vi "ElevatorPIDFinalPlat.vi"(9 "Elevator Setpoint":dbl format="%.2f") -> (15 "At Setpoint":bool)   [LabVIEW 2014]
uses:
  Robot Global Data.vi
  <vilib>/addons/control/pid/pid.llb/PID (DBL).vi
  <vilib>/addons/control/pid/NI_PID_pid.lvlib
panel:
  out "Encoder Graph":dbl[](graph)
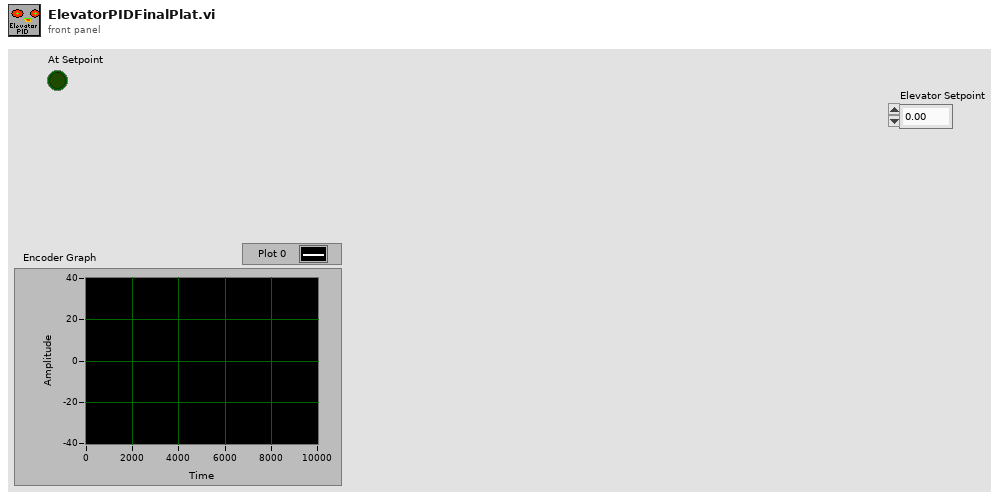
[diagram p1: front panel]
types:
  T1 = cluster{"proportional gain (Kc)":dbl, "integral time (Ti, min)":dbl, "derivative time (Td, min)":dbl}
  T2 = typedef "WPI_MotorControlDeviceRef.ctl" = cluster{"DeviceStatus":errorcluster, "Type":T3, "PWM":cluster{"Controller":T4, "PWM Channel":T5, "DeadBand":T6}, "CAN":cluster{"Device Number":u8, "Control Mode":T7, "Semaphore":T8, "Max Vout":dbl, "TalonSRX Control Mode":T9}, "Invert":bool, "TransformRef":T10, "InvTransformRef":T10}
  T3 = typedef "WPI_MotorControlType.ctl" = enum16{"PWM", "CAN", "CANTalonSRX"}
  T4 = typedef "FPGA_TypedefDigitalModule.ctl" = enum16{"Controller 1"}
  T5 = typedef "FPGA_DIOPWMChannel.ctl" = enum8{"PWM 0", "PWM 1", "PWM 2", "PWM 3", "PWM 4", "PWM 5", "PWM 6", "PWM 7", "PWM 8", "PWM 9", "PWM MXP 0", "PWM MXP 1", "PWM MXP 2", "PWM MXP 3", "PWM MXP 4", "PWM MXP 5", "PWM MXP 6", "PWM MXP 7", "PWM MXP 8", "PWM MXP 9", "Invalid"}
  T6 = typedef "WPI_PWMDeadband.ctl" = cluster{"Name":string, "maxPositivePwm":i32, "minPositivePwm":i32, "centerPwm":i32, "maxNegativePwm":i32, "minNegativePwm":i32, "angularRange":u16}
  T7 = typedef "WPI_CANJaguar_ControlMode.ctl" = enum8{"Percent VBus", "Current", "Speed", "Position", "Voltage"}
  T8 = typedef "Semaphore RefNum" = refnum<k1>
  T9 = typedef "WPI_CANTalonSRX_APIControlMode.ctl" = enum8{"Percent VBus", "Speed", "Position", "Slave", "Unchanged / Invalid"}
  T10 = typedef "WPI_PWMTransform_ConPane.ctl" = refnum<vi>
  T11 = typedef "WPI_CANTalonSRX_GlobalStatus.ctl" = cluster{"Applied Throttle":dbl, "Module Enabled":bool, "CAN Error":errorcluster, "Closed Loop Error":dbl, "Forward Limit Switch Closed":bool, "Reverse Limit Switch Closed":bool, "Sensor Position":dbl, "Sensor Velocity":dbl, "Current":dbl, "Sticky Fault - Over Temp":bool, "Sticky Fault - Under Voltage":bool, "Sticky Fault - Forward Limit":bool, "Sticky Fault - Reverse Limit":bool, "Sticky Fault - Forward Soft Limit":bool, "Sticky Fault - Reverse Soft Limit":bool, "Brake is Enabled":bool, "Encoder Position":dbl, "Encoder Velocity":dbl, "Encoder Index Count":dbl, "Encoder A Pin State":bool, "Encoder B Pin State":bool, "Encoder Index Pin State":bool, "Analog In":dbl, "Analog In Velocity":dbl, "Temperature (C)":dbl, "Battery Voltage":dbl}
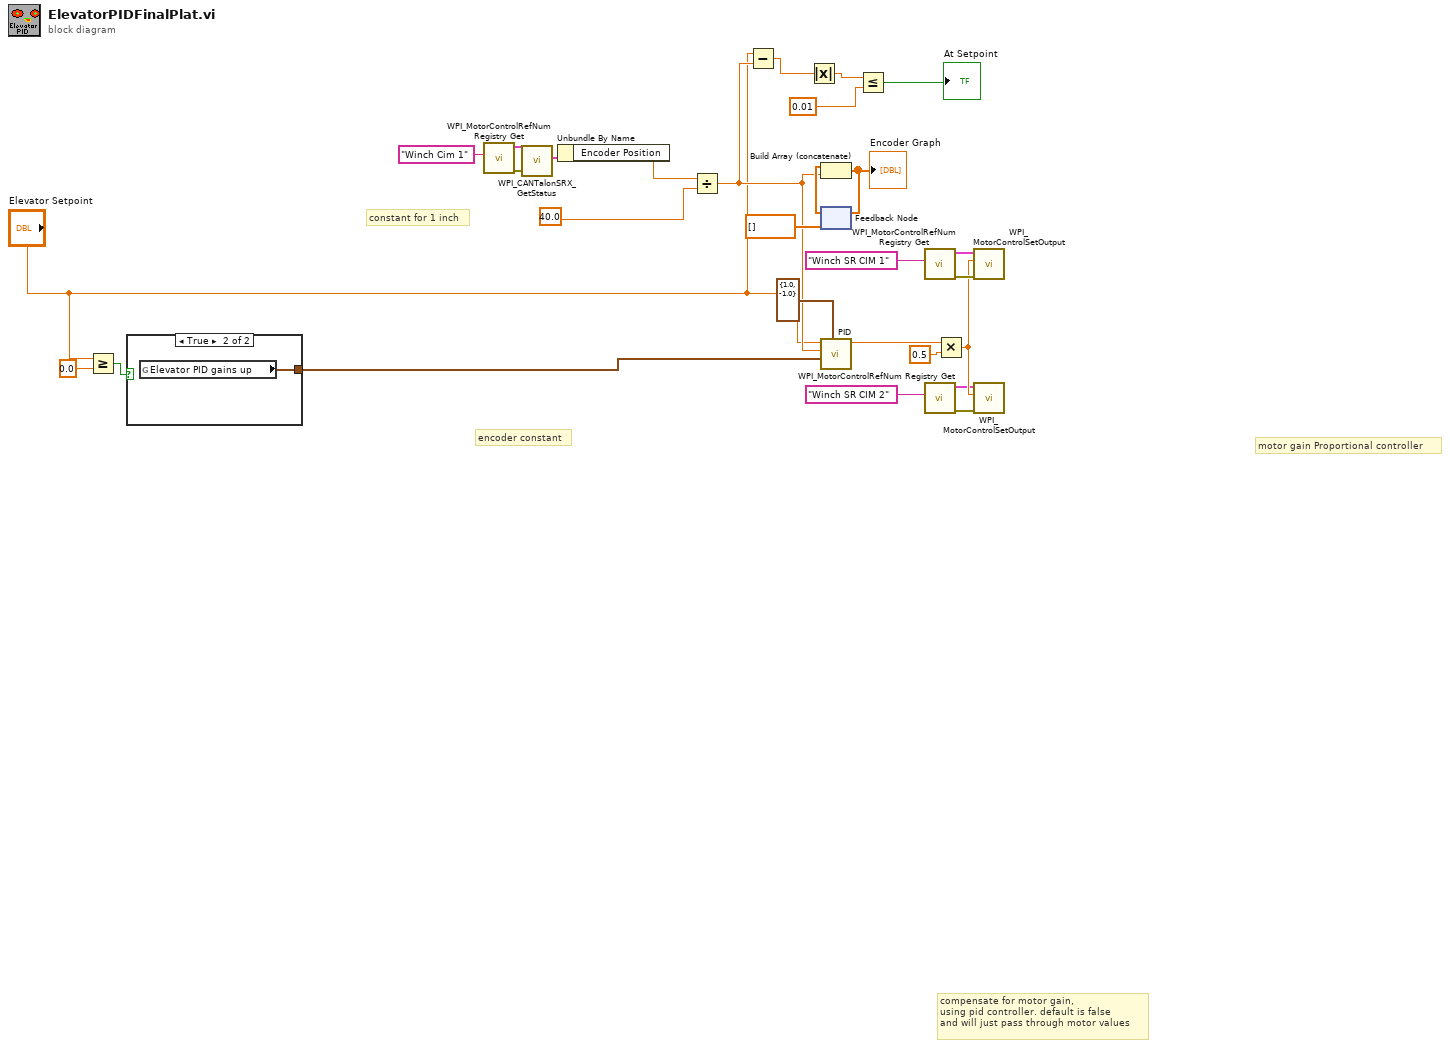
[diagram p0: block diagram]
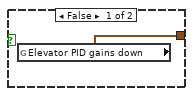
[diagram p2: hidden frame]
diagram:
  # "constant for 1 inch"
  # "encoder constant"
  # "motor gain Proportional controller"
  # "compensate for motor gain,\nusing pid controller. default is false\nand will just pass through motor values"
  n1 = Greater Or Equal?(x="Elevator Setpoint", y=0.0) -> (x >= y?=w16:bool)
  n2 = case shown="True" w16 {
    tunnel: [w29 w30] -> w27
    frame False {
      n3 = global read "Robot Global Data.vi" "Elevator PID gains down"() -> (w29:T1)
    }
    frame True {
      n4 = global read "Robot Global Data.vi" "Elevator PID gains up"() -> (w30:T1)
    }
  }
  n5 = call <vilib>:"WPI_MotorControlRefNum Registry Get.vi"("refnum name"="Winch Cim 1") -> ("error out"=w5:errorcluster, "MotorControlDevRef"=w4:T2)  [unwired: 9 in]
  n6 = call <vilib>:"WPI_CANTalonSRX_GetStatus.vi"("error in (no error)"=w5, "CAN Talon SRX Ref"=w4) -> ("Talon SRX Status"=w2:T11)  [unwired: 7 in, 2 out]
  n7 = Unbundle By Name(w2) -> ("Encoder Position"=w1:dbl)
  n8 = Divide(x=w1, y=40.0) -> (x/y=w14:dbl)
  n9 = Subtract(x="Elevator Setpoint", y=w14) -> (x-y=w12:dbl)
  n10 = Absolute Value(x=w12) -> (abs(x)=w11:dbl)
  n11 = feedback #1(dbl[] []) -> (w25:dbl[])
  n12 = Build Array (concatenate)(w25, w14) -> (w26:dbl[])
  "Encoder Graph" <- w26
  n13 = feedback-in #1(w26) -> ()
  n14 = call-poly <vilib>:"PID.vi"("output range"=cluster{"output high":dbl, "output low":dbl} {"output high"=1.0, "output low"=-1.0}, "PID gains"=w27, "process variable"=w14, "setpoint"="Elevator Setpoint") -> ("output"=w18:dbl)  [unwired: 6 in, 1 out]
  n15 = Less Or Equal?(x=w11, y=0.01) -> (x <= y?=→"At Setpoint":bool)
  n16 = call <vilib>:"WPI_MotorControlRefNum Registry Get.vi"("refnum name"="Winch SR CIM 1") -> ("error out"=w22:errorcluster, "MotorControlDevRef"=w21:T2)  [unwired: 9 in]
  n17 = call <vilib>:"WPI_MotorControlRefNum Registry Get.vi"("refnum name"="Winch SR CIM 2") -> ("error out"=w7:errorcluster, "MotorControlDevRef"=w6:T2)  [unwired: 9 in]
  n18 = Multiply(x=w18, y=0.5) -> (x*y=w20:dbl)
  n19 = call <vilib>:"WPI_MotorControlSetOutput.vi"("error in (no error)"=w22, "Output"=w20, "MotorControlDevRef"=w21) -> ()  [unwired: 6 in, 3 out]
  n20 = call <vilib>:"WPI_MotorControlSetOutput.vi"("error in (no error)"=w7, "Output"=w20, "MotorControlDevRef"=w6) -> ()  [unwired: 6 in, 3 out]
